vi "ge_SelRows.vi"(8 "error in":errorcluster, 10 "ChanGrp.lvclass":refnum<class "ChanGrp.lvclass">, 11 "Table Ref":refnum<vi>) -> (0 "error out":errorcluster, 2 "Selected Rows":i32[](array[numeric]))   [LabVIEW 2018]
uses:
  Classes/Cfg Grandmaster/Class Chan Group/ChanGrp.lvclass
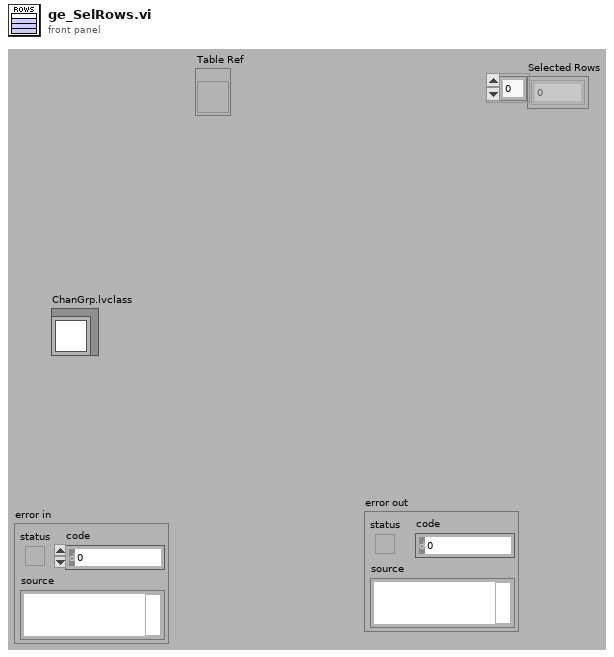
[diagram p1: front panel]
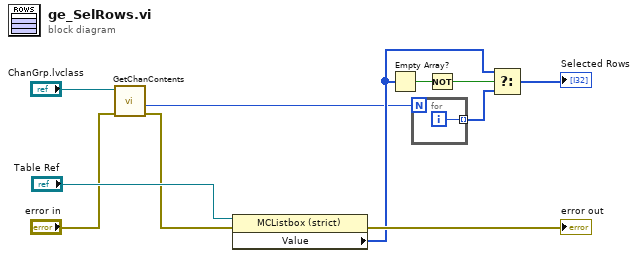
[diagram p0: block diagram]
diagram:
  n1 = call "GetChanContents.vi"("error in"="error in", "ChanGrp.lvclass"="ChanGrp.lvclass") -> ("error out"=w1:errorcluster, "Num of Chans"=w3:i32)  [unwired: 3 in, 5 out]
  n2 = property on="Property Node" class="MCListbox (strict)"(reference="Table Ref", error in=w1) -> (error out=→"error out":errorcluster, "Value"=w9:i32[])  [unwired: 1 out]
  n3 = Empty Array?(array=w9) -> (empty?=w6:bool)
  n4 = for {
    N: w3 -> [_]
    tunnel: [w12] -> w8 mode=indexing
    i -> [w12]
  }
  n5 = Not(x=w6) -> (.not. x?=w7:bool)
  n6 = Select(t=w9, s=w7, f=w8) -> (s? t:f=→"Selected Rows":i32[])
